vi "one_measurement.vi"(6 "Rsh, Ohm":dbl=98.2 format="%0.1f", 8 "Error (in)":errorcluster, 9 "Number of points":i32=100, 10 "time for one scan, ms":u32=100, 11 "DAQ AI task (in)":refnum<k21>) -> (0 "Error (out)":errorcluster, 1 "Data":T1, 3 "DAQ AI task (out)":refnum<k21>)   [LabVIEW 2017]
uses:
  <vilib>/DAQmx/read.llb/DAQmx Read (Analog 1D Wfm NChan NSamp).vi
  <vilib>/DAQmx/miscellaneous.llb/DAQmx Fill In Error Info.vi
panel:
  out "size of buffer":i32=9984
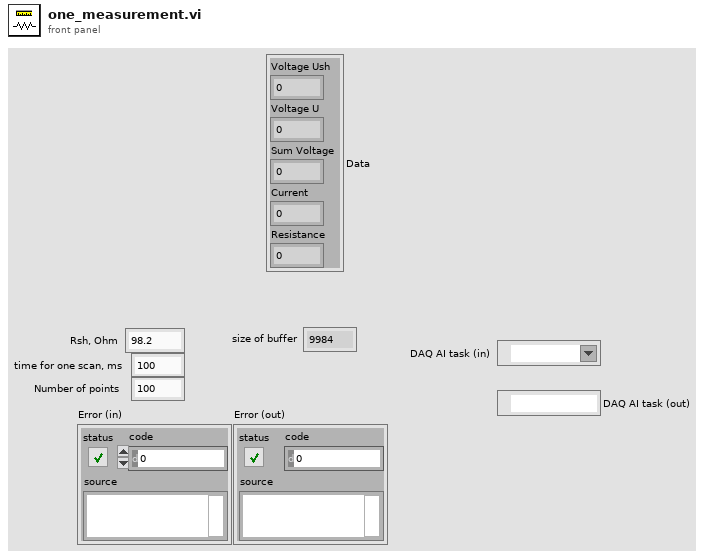
[diagram p1: front panel]
types:
  T1 = cluster{"Voltage Ush":dbl, "Voltage U":dbl, "Sum Voltage":dbl, "Current":dbl, "Resistance":dbl}
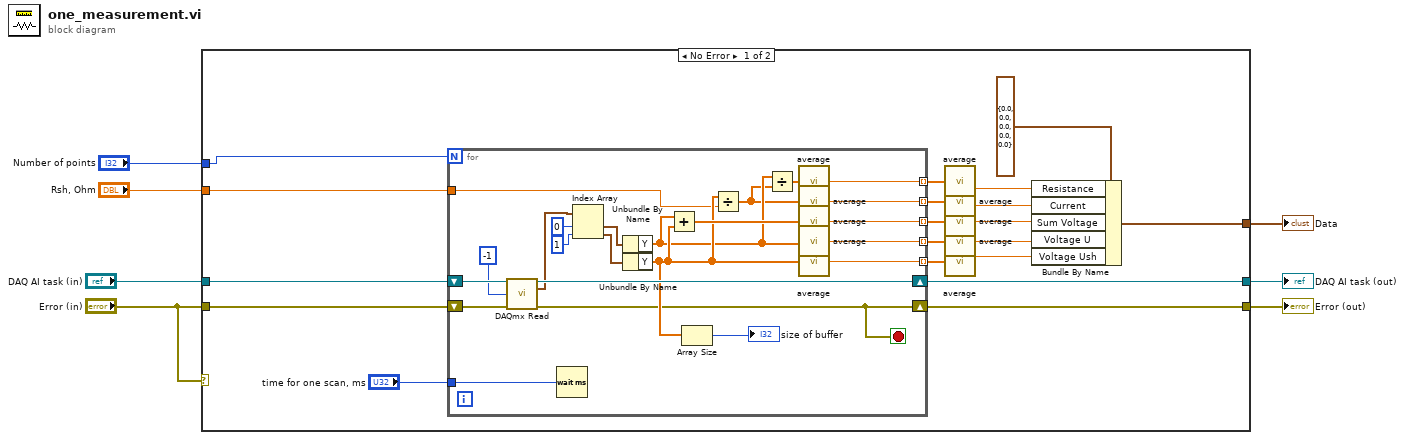
[diagram p0: block diagram]
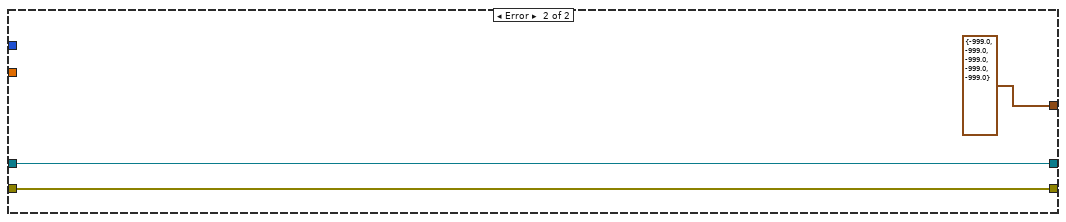
[diagram p2: hidden frame]
diagram:
  n1 = case shown="No Error" "Error (in)" {
    tunnel: "DAQ AI task (in)" -> [w26 w52]
    tunnel: "Error (in)" -> [w25 w51]
    tunnel: [w23 w52] -> w6
    tunnel: [w22 w51] -> w5
    tunnel: [w10 T1 {"Voltage Ush"=-999.0, "Voltage U"=-999.0, "Sum Voltage"=-999.0, "Current"=-999.0, "Resistance"=-999.0} ("Cluster")] -> w3
    tunnel: "Rsh, Ohm" -> [w9 _]
    tunnel: "Number of points" -> [w8 _]
    frame No Error {
      n2 = for {
        N: w8 -> [_]
        tunnel: "time for one scan, ms" -> [w33]
        shift-right: [w34] -> w22
        shift-left: w25 -> [w47]
        shift-right: [w46] -> w23
        shift-left: w26 -> [w49]
        tunnel: [w32] -> w21 mode=indexing
        tunnel: [w31] -> w20 mode=indexing
        tunnel: [w30] -> w19 mode=indexing
        tunnel: [w29] -> w18 mode=indexing
        tunnel: [w28] -> w17 mode=indexing
        tunnel: w9 -> [w27]
        stop <- w34 stop-if-true
        n3 = call-poly <vilib>:"DAQmx Read.vi"("task/channels in"=w49, "number of samples per channel"=-1, "error in"=w47) -> ("task out"=w46:refnum<k21>, "data"=w45:waveform(dbl)[], "error out"=w34:errorcluster)  [unwired: 10 in]
        n4 = Wait (ms)(milliseconds to wait=w33) -> ()  [unwired: 1 out]
        n5 = Index Array(array=w45, index #1=0 ("index"), index #2=1 ("index")) -> (element #1=w42:waveform(dbl), element #2=w41:waveform(dbl))
        n6 = Unbundle By Name(w42) -> ("Y"=w38:dbl[])
        n7 = Unbundle By Name(w41) -> ("Y"=w39:dbl[])
        n8 = Add(x=w38, y=w39) -> (x+y=w40:dbl[])
        n9 = Array Size(array=w39) -> (size(s)=→"size of buffer":i32)
        n10 = Divide(x=w39, y=w27) -> (x/y=w37:dbl[])
        n11 = Divide(x=w38, y=w37) -> (x/y=w36:dbl[])
        n12 = call "average.vi"("Array"=w36) -> ("Average"=w32:dbl)
        n13 = call "average.vi"("Array"=w37) -> ("Average"=w31:dbl)
        n14 = call "average.vi"("Array"=w40) -> ("Average"=w30:dbl)
        n15 = call "average.vi"("Array"=w38) -> ("Average"=w29:dbl)
        n16 = call "average.vi"("Array"=w39) -> ("Average"=w28:dbl)
      }
      n17 = call "average.vi"("Array"=w21) -> ("Average"=w15:dbl)
      n18 = call "average.vi"("Array"=w20) -> ("Average"=w14:dbl)
      n19 = call "average.vi"("Array"=w19) -> ("Average"=w13:dbl)
      n20 = call "average.vi"("Array"=w18) -> ("Average"=w12:dbl)
      n21 = call "average.vi"("Array"=w17) -> ("Average"=w11:dbl)
      n22 = Bundle By Name(cluster=T1 {"Voltage Ush"=0.0, "Voltage U"=0.0, "Sum Voltage"=0.0, "Current"=0.0, "Resistance"=0.0} ("Cluster"), "Resistance"=w15, "Current"=w14, "Sum Voltage"=w13, "Voltage U"=w12, "Voltage Ush"=w11) -> (w10:T1)
    }
    frame Error {
    }
  }
  "DAQ AI task (out)" <- w6
  "Error (out)" <- w5
  "Data" <- w3
